vi "Servo_SetAngle.vi"(8 "error in":errorcluster, 9 "Angle in":dbl min=-45.0 max=45.0, 10 "PWM":T1=1 items=["Invalid"=0, "PWM1"=1, "PWM2"=2, "PWM9"=9, "PWM10"=10]) -> (0 "error out":errorcluster, 2 "Angle out":dbl)   [LabVIEW 2009, in "Servo.lvlib"]
doc: "A function for setting the angle for some particular servo. It takes an angle and the servo to be set as input. The input ranges between -45 and 45deg. \n\nThe function scales the input to the right PWM signal (assuming that the servo need to be feed a signal with the period of 20000 uSec).\n\nNote: Before using this function you will need to initialise the servo and enable it to send to PWM, this is done by calling the Servo_init function once at the start. Also uses a reference to the FPGA."
uses:
  Servo.lvlib
  PWM/PWM_Name.ctl
  PWM.lvlib
panel:
  out "High out":u32
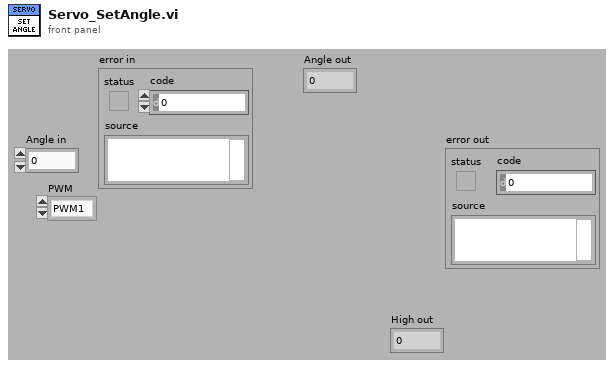
[diagram p1: front panel]
types:
  T1 = typedef "PWM.lvlib/PWM_Name.ctl" = u16
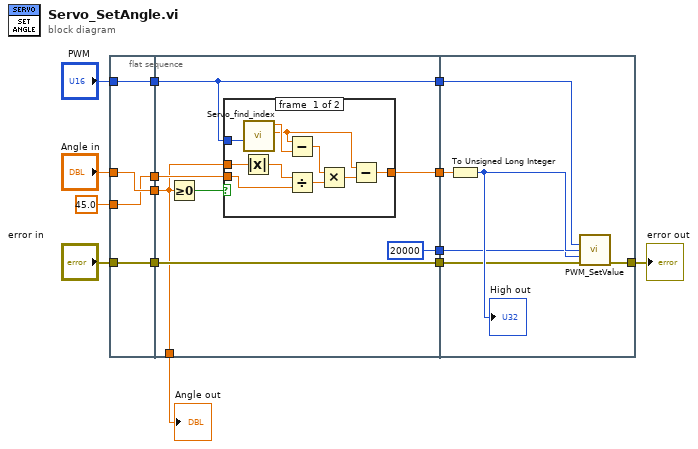
[diagram p0: block diagram]
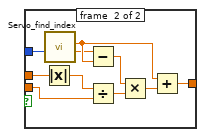
[diagram p2: hidden frame]
diagram:
  n1 = flat-sequence {
    tunnel: "PWM" -> [w17]
    tunnel: "Angle in" -> [w18]
    tunnel: [w18] -> w14
    tunnel: [w17] -> w13
    tunnel: 45.0 ("y") -> [w16]
    tunnel: [w16] -> w12
    tunnel: "error in" -> [w15]
    tunnel: [w15] -> w11
    tunnel: w14 -> [w19]
    tunnel: w13 -> [w20]
    tunnel: [w24] -> w10
    tunnel: w12 -> [w23]
    tunnel: [u32 20000 ("Period (uSec)")] -> w9
    tunnel: [w21] -> w8
    tunnel: w11 -> [w21]
    tunnel: [w20] -> w7
    tunnel: [w19] -> w1
    tunnel: w10 -> [w51]
    tunnel: w9 -> [w49]
    tunnel: w8 -> [w48]
    tunnel: [w47] -> w4
    tunnel: w7 -> [w46]
    frame #0 {
    }
    frame #1 {
      n2 = Greater Or Equal To 0?(x=w19) -> (x >= 0?=w25:bool)
      n3 = case shown="True" w25 {
        tunnel: w19 -> [w34 w44]
        tunnel: w20 -> [w35 w45]
        tunnel: [w31 w39] -> w24
        tunnel: w23 -> [w27 w41]
        frame #0 {
          n4 = Absolute Value(x=w34) -> (abs(x)=w28:dbl)
          n5 = call "Servo_find_index.vi"("PWM"=w35) -> ("0 deg"=w29:dbl, "-45 deg"=w32:dbl)  [unwired: 7 in, 2 out]
          n6 = Subtract(x=w29, y=w32) -> (x-y=w33:dbl)
          n7 = Divide(x=w28, y=w27) -> (x/y=w26:dbl)
          n8 = Multiply(x=w33, y=w26) -> (x*y=w30:dbl)
          n9 = Subtract(x=w29, y=w30) -> (x-y=w31:dbl)
        }
        frame #1 {
          n10 = Absolute Value(x=w44) -> (abs(x)=w42:dbl)
          n11 = call "Servo_find_index.vi"("PWM"=w45) -> ("45 deg"=w36:dbl, "0 deg"=w37:dbl)  [unwired: 7 in, 2 out]
          n12 = Subtract(x=w36, y=w37) -> (x-y=w43:dbl)
          n13 = Divide(x=w42, y=w41) -> (x/y=w40:dbl)
          n14 = Multiply(x=w43, y=w40) -> (x*y=w38:dbl)
          n15 = Add(x=w37, y=w38) -> (x+y=w39:dbl)
        }
      }
    }
    frame #2 {
      n16 = To Unsigned Long Integer(number=w51) -> (unsigned 32bit integer=w50:u32)
      "High out" <- w50
      n17 = call "PWM_SetValue.vi"("PWM"=w46, "High (uSec)"=w50, "Period (uSec)"=w49, "error in"=w48) -> ("error out"=w47:errorcluster)  [unwired: 11 in]
    }
  }
  "error out" <- w4
  "Angle out" <- w1
